vi "PH_DeformableMirror.panel.vi"(0 "object ref":refnum<vi>, 5 "error in (no error)":errorcluster) -> (19 "error out":errorcluster)   [LabVIEW 2014, in "PH_DeformableMirror.lvlib"]
doc: "By this VI a ross relais can be monitored and switched. \n\nThe indicators \"CLOSED\", \"OPEN\" and \"SWITCH STATE\" show the value of the Beckhoff-Tag: blue indicates bad tag status reference problems, darkgreen false and lightgreen on. If everything is working fine, \"CLOSED\" and \"SWITCH STATE\" should show the same value, while \"OPEN\" has the opposite value. \n\nThe oval button switches the ross relais. It should be in the same state as the \"SWITCH STATE\" indicator. \n\n\"EXIT\" closes the front panel (GUI), while \"Delete Instance\" disconnects and removes the instance from the PCS.\n\nThis VI has no machine safety relevant logig: there is neither a check of internal conclict nor with other objects, for example conflict with other ross relais. Therefore it must be handled with care and should be operated by well educated operators only. It is forseen exclusively for direct operating and testing of the system. \n\nLicense Agreement for this software:\n\nCopyright (C)\nGesellschaft für Schwerionenforschung, GSI\nPlanckstr. 1\n64291 Darmstadt\nGermany\n\nContact: D.Beck@gsi.de \n\nThis program is free software; you can redistribute it and/or modify it under the terms of the GNU General Public License as published by the Free Software Foundation; either version 2 of the license, or (at your option) any later version.\n\nThis program is distributed in the hope that it will be useful, but WITHOUT ANYW ARRANTY; without even the implied warranty of MERCHANTABILITY or FITNESS FOR A PARTICULAR PURPOSE. See the GNU General License for more details (http://www.gnu.org).\n\nGesellschaft für Schwerionenforschung, GSI\nPlanckstr. 1, 64291 Darmstadt, Germany\nFor all questions and ideas contact: M.Richter@gsi.de, H.Brand@gsi.de or D.Beck@gsi.de.\nLast update: 18-DEC-2002"
uses:
  PH_DeformableMirror.lvlib
  PH_StatusHandler/PH_StatusHandler.GUI element.ctl
  CSCore/CSObj/CSObj.lvlib
  PH_Common/PH_Common.lvlib
  CSCore/CSSystem/CSSystemLib/CSSystemLib.lvlib
  PH_Class/PH_Class.lvlib
  PH_StatusHandler/PH_StatusHandler.lvlib
panel:
  in  "Hysteresis\nCompensation?":bool
  in  "Set all Zero":bool
  in  "Channel Voltages [V]":dbl[](array[numeric])
  in  "Set all Channels":bool
  in  "Voltage [V]":dbl
  in  "Channel":u32
  in  "Set Channel":bool
  in  "HV on":bool
  out "Device Error":errorcluster
  out "Status":T1
  in  "Delete":bool
  in  "Exit":bool
  # "PCS"
  # "3.40"
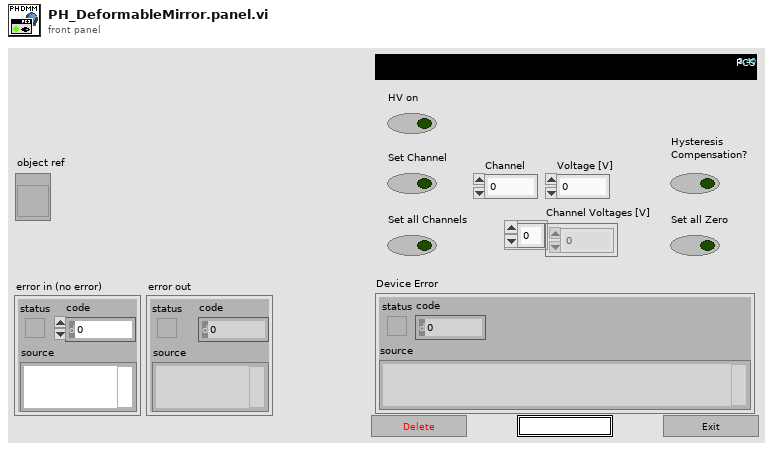
[diagram p1: front panel]
types:
  T1 = typedef "PH_StatusHandler.lvlib/PH_StatusHandler.GUI element.ctl" = u16
  T2 = typedef "PH_DeformableMirror.lvlib/PH_DeformableMirror.i attribute.ctl" = cluster{"DMirror.lvlib:DMirrorBase.lvclass":refnum<class "DMirrorBase.lvclass">, "Device error":errorcluster, "GUI Refs":cluster{"Delete":refnum<vi>, "Device Error":refnum<vi>, "HV on":refnum<vi>, "Channel":refnum<vi>, "Voltage":refnum<vi>, "Channel Voltages":refnum<vi>}}
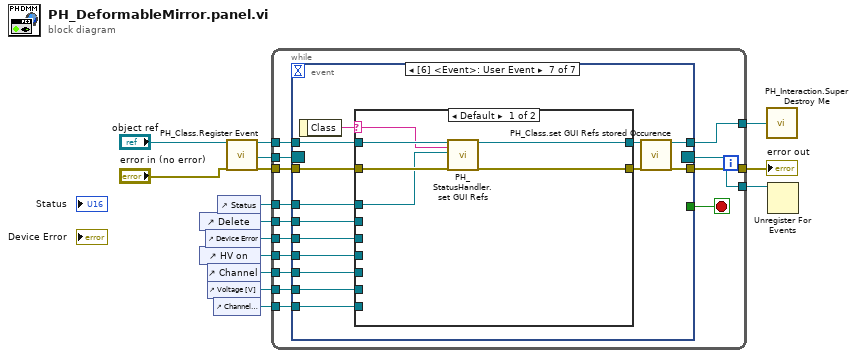
[diagram p0: block diagram]
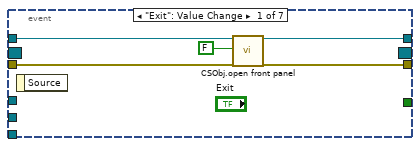
[diagram p2: hidden frame]
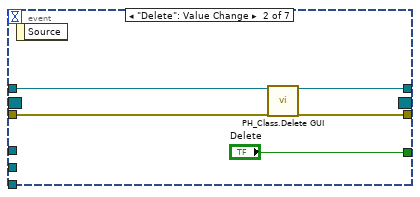
[diagram p3: hidden frame]
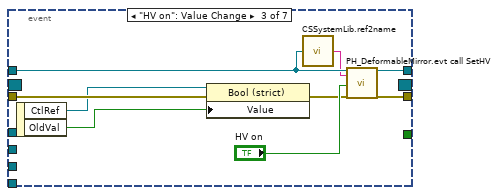
[diagram p4: hidden frame]
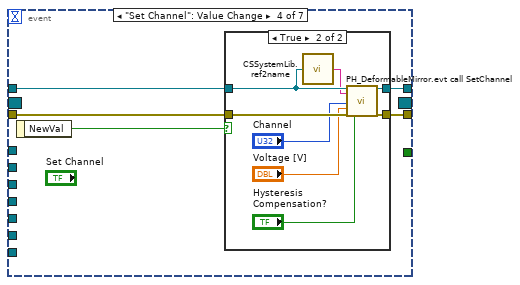
[diagram p5: hidden frame]
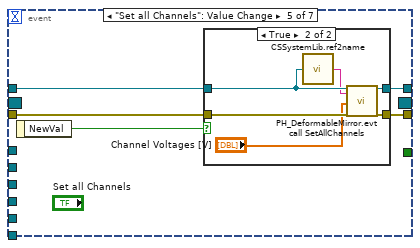
[diagram p7: hidden frame]
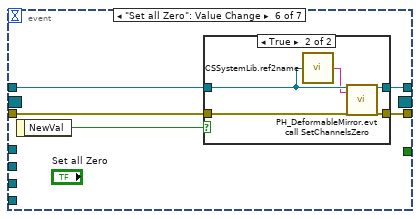
[diagram p9: hidden frame]
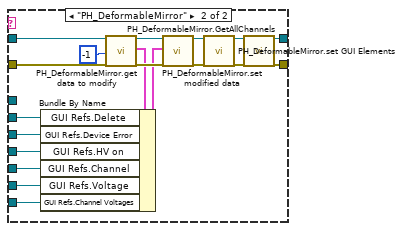
[diagram p11: hidden frame]
diagram:
  n1 = control-ref of="Delete"() -> (w6:refnum<vi>)
  n2 = control-ref of="HV on"() -> (w4:refnum<vi>)
  n3 = control-ref of="Device Error"() -> (w5:refnum<vi>)
  n4 = control-ref of="Channel"() -> (w3:refnum<vi>)
  n5 = control-ref of="Voltage [V]"() -> (w2:refnum<vi>)
  n6 = control-ref of="Channel Voltages [V]"() -> (w1:refnum<vi>)
  n7 = control-ref of="Status"() -> (w7:refnum<vi>)
  n8 = call "PH_Class.Register Event.vi"("i ref in"="object ref", "error in (no error)"="error in (no error)") -> ("i ref out"=w13:refnum<vi>, "Event Registration Refnum"=w11:refnum<event-registration>, "error out"=w12:errorcluster)  [unwired: 15 in]
  n9 = while {
    tunnel: w13 -> [w26]
    tunnel: [w25] -> w15
    tunnel: w12 -> [w28]
    tunnel: [w27] -> w14
    tunnel: w11 -> [w24]
    tunnel: [w23] -> w10
    tunnel: w7 -> [w22]
    tunnel: w6 -> [w21]
    tunnel: w5 -> [w20]
    tunnel: w4 -> [w19]
    tunnel: w3 -> [w18]
    tunnel: w2 -> [w17]
    tunnel: w1 -> [w16]
    stop <- w29 stop-if-true
    n10 = event shown="[6] <Event>: User Event" {
      selector: w24 -> [_ _ _ _ _ _ _]
      dyn-events: [_ _ _ _ _ _ _] -> w23
      timeout: _ -> [_ _ _ _ _ _ _]
      tunnel: [_ "Delete" _ _ _ _ _] -> w29
      tunnel: w26 -> [w34 w38 w44 w51 w66 w79 w98]
      tunnel: w28 -> [w32 w37 w48 w50 w65 w78 w97]
      tunnel: [w31 w36 w47 w53 w68 w81 w101] -> w27
      tunnel: [w30 w35 w46 w52 w67 w80 w102] -> w25
      tunnel: w22 -> [_ _ _ _ _ _ w95]
      tunnel: w21 -> [_ _ _ _ _ _ w94]
      tunnel: w20 -> [_ _ _ _ _ _ w93]
      tunnel: w19 -> [_ _ _ _ _ _ w92]
      tunnel: w18 -> [_ _ _ _ _ _ w91]
      tunnel: w17 -> [_ _ _ _ _ _ w90]
      tunnel: w16 -> [_ _ _ _ _ _ w89]
      event "Exit": Value Change {
        n11 = event-data() -> ()  [unwired: 1 in, 1 out]
        n12 = call "CSObj.open front panel.vi"("i ref in"=w34, "frontPanelOpen"=FALSE ("front panel open"), "error in (no error)"=w32) -> ("i ref out"=w30:refnum<vi>, "error out"=w31:errorcluster)  [unwired: 15 in]
      }
      event "Delete": Value Change {
        n13 = event-data() -> ()  [unwired: 1 in, 1 out]
        n14 = call "PH_Class.Delete GUI.vi"("VI in"=w38, "error in (no error)"=w37) -> ("VI out"=w35:refnum<vi>, "error out"=w36:errorcluster)  [unwired: 16 in]
      }
      event "HV on": Value Change {
        n15 = event-data() -> ("CtlRef"=w41:refnum<vi>, "OldVal"=w40:bool)  [unwired: 1 in]
        n16 = property class="Bool (strict)"(reference=w41, error in=w48, "Value"=w40) -> (error out=w42:errorcluster)  [unwired: 1 out]
        n17 = call "CSSystemLib.ref2name.vi"("obj refnum"=w44) -> ("name"=w43:string)
        n18 = call "PH_DeformableMirror.evt call SetHV.vi"("i ref in"=w44, "Object"=w43, "HV on/off"="HV on", "error in (no error)"=w42) -> ("i ref out"=w46:refnum<vi>, "error out"=w47:errorcluster)  [unwired: 14 in]
      }
      event "Set Channel": Value Change {
        n19 = event-data() -> ("NewVal"=w49:bool)  [unwired: 1 in]
        n20 = case shown="True" w49 {
          tunnel: [w54 w63] -> w53
          tunnel: [w55 w62] -> w52
          tunnel: w51 -> [w55 w61]
          tunnel: w50 -> [w54 w59]
          frame False {
          }
          frame True {
            n21 = call "CSSystemLib.ref2name.vi"("obj refnum"=w61) -> ("name"=w60:string)
            n22 = call "PH_DeformableMirror.evt call SetChannel.vi"("i ref in"=w61, "Object"=w60, "channel"="Channel", "voltage"="Voltage [V]", "error in (no error)"=w59, "Hysteresis Compensation? (false)"="Hysteresis\nCompensation?") -> ("i ref out"=w62:refnum<vi>, "error out"=w63:errorcluster)  [unwired: 12 in]
          }
        }
      }
      event "Set all Channels": Value Change {
        n23 = event-data() -> ("NewVal"=w64:bool)  [unwired: 1 in]
        n24 = case shown="True" w64 {
          tunnel: [w69 w76] -> w68
          tunnel: [w70 w75] -> w67
          tunnel: w66 -> [w70 w74]
          tunnel: w65 -> [w69 w72]
          frame False {
          }
          frame True {
            n25 = call "CSSystemLib.ref2name.vi"("obj refnum"=w74) -> ("name"=w73:string)
            n26 = call "PH_DeformableMirror.evt call SetAllChannels.vi"("i ref in"=w74, "Object"=w73, "Voltages"="Channel Voltages [V]", "error in (no error)"=w72) -> ("i ref out"=w75:refnum<vi>, "error out"=w76:errorcluster)  [unwired: 14 in]
          }
        }
      }
      event "Set all Zero": Value Change {
        n27 = event-data() -> ("NewVal"=w77:bool)  [unwired: 1 in]
        n28 = case shown="True" w77 {
          tunnel: [w82 w88] -> w81
          tunnel: [w83 w87] -> w80
          tunnel: w79 -> [w83 w86]
          tunnel: w78 -> [w82 w84]
          frame False {
          }
          frame True {
            n29 = call "CSSystemLib.ref2name.vi"("obj refnum"=w86) -> ("name"=w85:string)
            n30 = call "PH_DeformableMirror.evt call SetChannelsZero.vi"("i ref in"=w86, "Object"=w85, "error in (no error)"=w84) -> ("i ref out"=w87:refnum<vi>, "error out"=w88:errorcluster)  [unwired: 15 in]
          }
        }
      }
      event User Event {
        n31 = event-data() -> ("Class"=w96:string)  [unwired: 1 in]
        n32 = case shown="Default" w96 {
          selector: w96 -> [w103 _]
          tunnel: [w105 w127] -> w100
          tunnel: [w107 w126] -> w99
          tunnel: w98 -> [w106 w118]
          tunnel: w97 -> [w108 w116]
          tunnel: w95 -> [w104 _]
          tunnel: w94 -> [_ w114]
          tunnel: w93 -> [_ w113]
          tunnel: w92 -> [_ w112]
          tunnel: w91 -> [_ w111]
          tunnel: w90 -> [_ w110]
          tunnel: w89 -> [_ w109]
          frame Default {
            n33 = call "PH_StatusHandler.set GUI Refs.vi"("i ref in"=w106, "Class"=w103, "GUI Ref"=w104, "error in (no error)"=w108) -> ("i ref out"=w105:refnum<vi>, "error out"=w107:errorcluster)  [unwired: 14 in]
          }
          frame "PH_DeformableMirror" {
            n34 = call "PH_DeformableMirror.get data to modify.vi"("i ref in"=w118, "ms timeout (10000)"=-1, "error in (no error)"=w116) -> ("i ref out"=w123:refnum<vi>, "i attribute"=w121:T2, "error out"=w122:errorcluster)  [unwired: 13 in, 1 out]
            n35 = Bundle By Name(cluster=w121, "GUI Refs.Delete"=w114, "GUI Refs.Device Error"=w113, "GUI Refs.HV on"=w112, "GUI Refs.Channel"=w111, "GUI Refs.Voltage"=w110, "GUI Refs.Channel Voltages"=w109) -> (w120:T2)
            n36 = call "PH_DeformableMirror.set modified data.vi"("i ref in"=w123, "i attribute"=w120, "error in (no error)"=w122) -> ("i ref out"=w117:refnum<vi>, "error out"=w115:errorcluster)  [unwired: 15 in]
            n37 = call "PH_DeformableMirror.set GUI Elements.vi"("VI in"=w117, "error in (no error)"=w115) -> ("VI out"=w124:refnum<vi>, "error out"=w125:errorcluster)  [unwired: 16 in]
            n38 = call "PH_DeformableMirror.GetAllChannels.vi"("VI in"=w124, "error in (no error)"=w125) -> ("VI out"=w127:refnum<vi>, "error out"=w126:errorcluster)  [unwired: 16 in]
          }
        }
        n39 = call "PH_Class.set GUI Refs stored Occurence.vi"("i ref in"=w100, "error in (no error)"=w99) -> ("i ref out"=w102:refnum<vi>, "error out"=w101:errorcluster)  [unwired: 16 in]
      }
    }
  }
  "error out" <- w14
  n40 = call "PH_Interaction.Super Destroy Me.vi"("i ref out"=w15) -> ()
  n41 = Unregister For Events(event registration refnum=w10) -> ()  [unwired: 1 in, 1 out]
